vi "Close.vi"(8 "error in":errorcluster, 11 "VISA resource name":refnum<visa-resource-name>) -> (0 "error out":errorcluster)   [LabVIEW 2021, in "Keysight U1282A.lvlib"]
doc: "Este bloque cierra la interfaz de comunicación serial (VISA) del instrumento U1282A."
uses:
  Keysight U1282A.lvlib
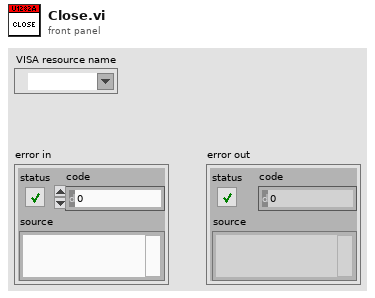
[diagram p1: front panel]
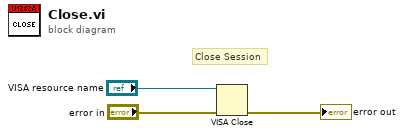
[diagram p0: block diagram]
diagram:
  # "Close Session"
  n1 = VISA Close(VISA resource name="VISA resource name", error in (no error)="error in") -> (error out=→"error out":errorcluster)
